vi "CreateWiringsNode.vi"(7 "DOM Document":refnum<k20>, 8 "Error In":errorcluster, 11 "Wirings":T1[](array[typedef])) -> (0 "Error Out":errorcluster, 3 "Wirings Node":refnum<k20>)   [LabVIEW 2013]
uses:
  driver/Public/Controls/SMUSense.ctl
  libs/LV-Utilities/LV-Utilities.lvlib
  driver/Keithley-2602.lvlib
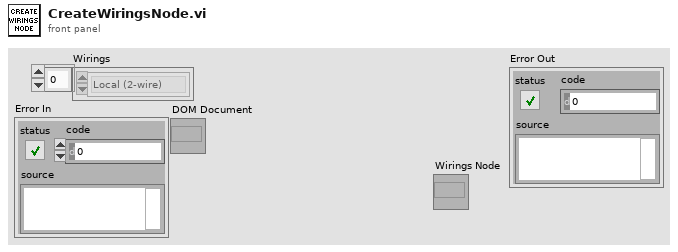
[diagram p1: front panel]
types:
  T1 = typedef "Keithley-2602.lvlib/SMUSense.ctl" = enum16{"Local (2-wire)", "Remote (4-wire)", "Calibration"}
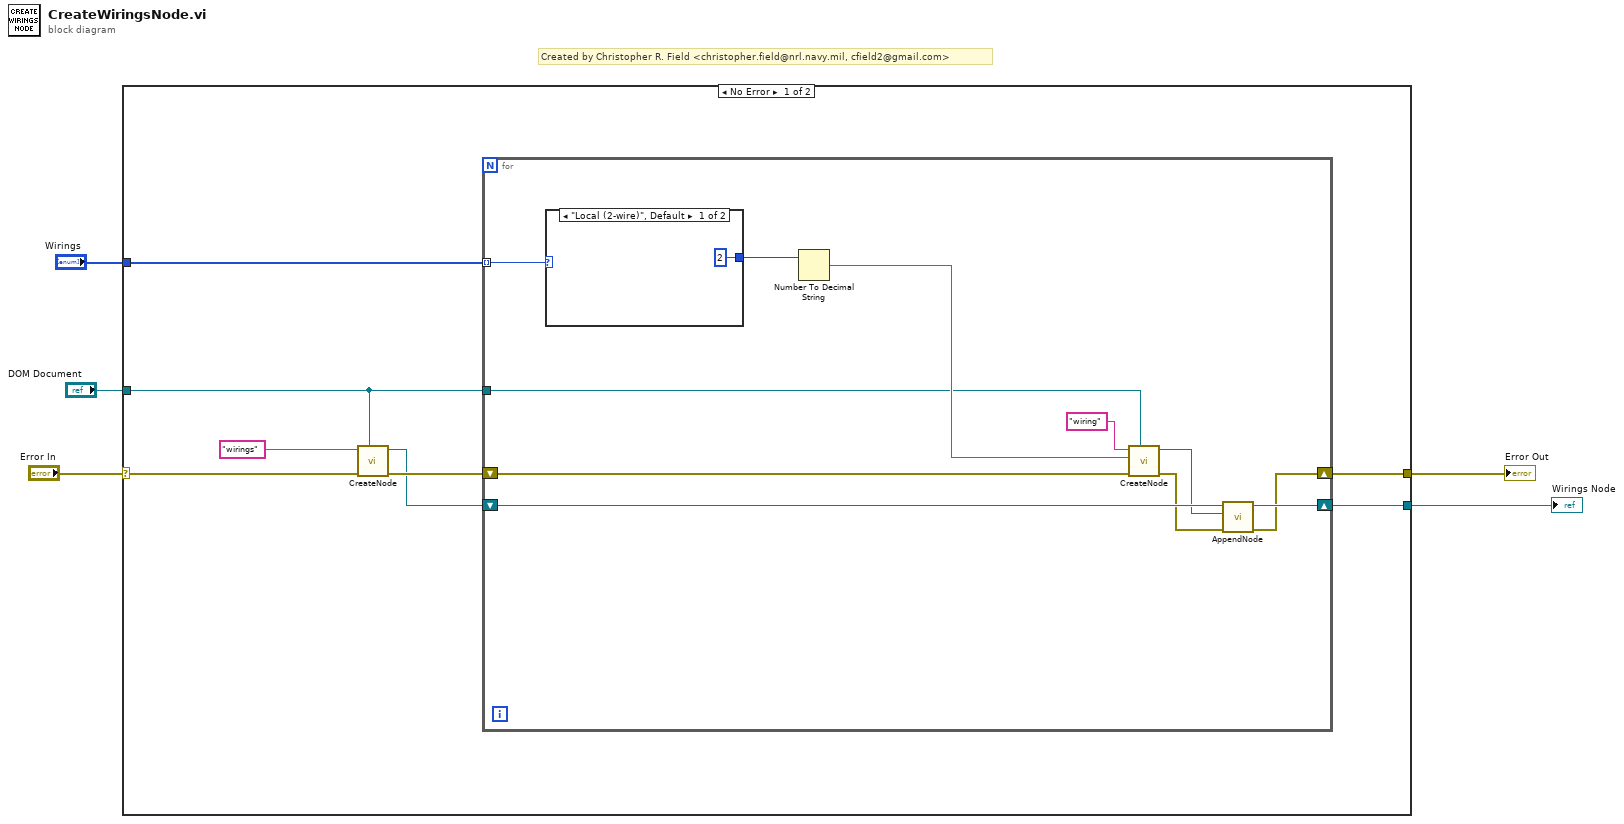
[diagram p0: block diagram]
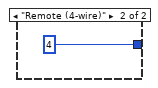
[diagram p2: hidden frame]
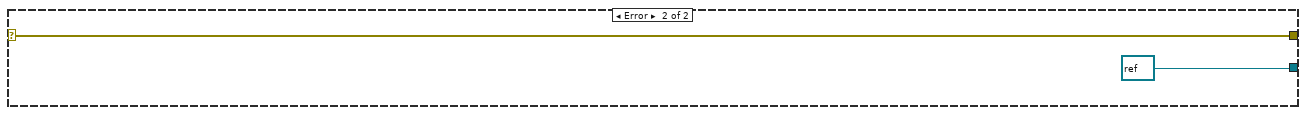
[diagram p3: hidden frame]
diagram:
  # "Created by Christopher R. Field <christopher.field@nrl.navy.mil, cfield2@gmail.com>"
  n1 = case shown="No Error" "Error In" {
    selector: "Error In" -> [w9 w28]
    tunnel: "Wirings" -> [w13 _]
    tunnel: "DOM Document" -> [w6 _]
    tunnel: [w12 refnum<k20> refnum ("Wirings Node 2")] -> w2
    tunnel: [w11 w28] -> w1
    frame No Error {
      n2 = call "CreateNode.vi"("DOM Document"=w6, "Error In"=w9, "Tag Name"="wirings") -> ("Error out"=w10:errorcluster, "Node"=w7:refnum<k20>)  [unwired: 7 in]
      n3 = for {
        shift-right: [w16] -> w11
        shift-left: w10 -> [w24]
        tunnel: w13 -> [w23] mode=indexing
        shift-right: [w18] -> w12
        shift-left: w7 -> [w19]
        tunnel: w6 -> [w14]
        n4 = case shown="\"Local (2-wire)\", Default" w23 {
          tunnel: [2 4] -> w22
          frame "Local (2-wire)", Default {
          }
          frame "Remote (4-wire)" {
          }
        }
        n5 = Number To Decimal String(number=w22) -> (decimal integer string=w21:string)  [unwired: 1 in]
        n6 = call "CreateNode.vi"("DOM Document"=w14, "Error In"=w24, "Text"=w21, "Tag Name"="wiring") -> ("Error out"=w17:errorcluster, "Node"=w15:refnum<k20>)  [unwired: 6 in]
        n7 = call "AppendNode.vi"("Error In"=w17, "Child Node"=w15, "Parent Node In"=w19) -> ("Error Out"=w16:errorcluster, "Parent Node Out"=w18:refnum<k20>)  [unwired: 7 in]
      }
    }
    frame Error {
    }
  }
  "Wirings Node" <- w2
  "Error Out" <- w1
